vi "FG_registeredwindows.vi"(8 "error in (no error)":errorcluster, 10 "window":T2, 11 "action":T1) -> (0 "error out":errorcluster, 2 "windows":T2[](array[typedef]))   [LabVIEW 2009]
uses:
  child window props.ctl
  FG states.ctl
panel:
  in  "Error range offset":i32=5500
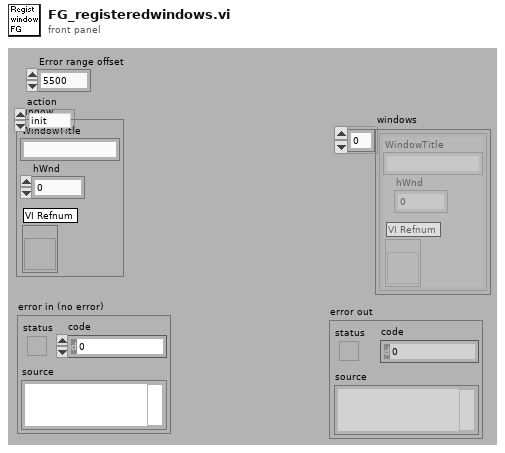
[diagram p1: front panel]
types:
  T1 = typedef "FG states.ctl" = enum16{"init", "add", "replace", "remove", "read"}
  T2 = typedef "child window props.ctl" = cluster{"WindowTitle":string, "hWnd":u32, "VI Refnum":refnum<vi>}
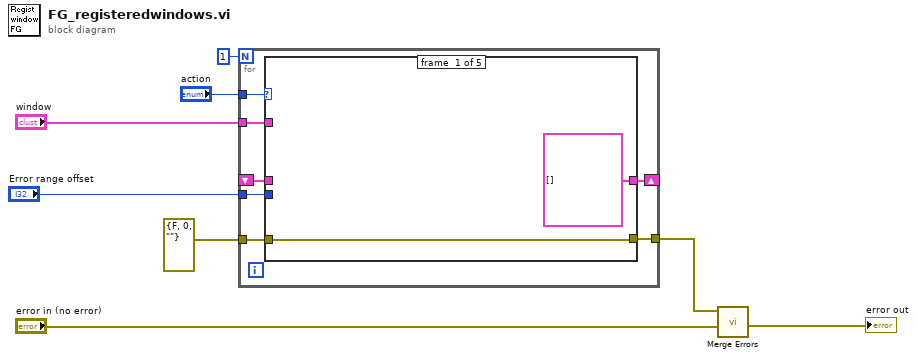
[diagram p0: block diagram]
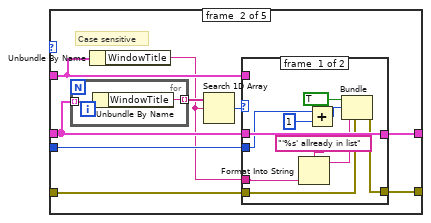
[diagram p2: hidden frame]
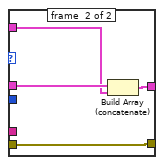
[diagram p3: hidden frame]
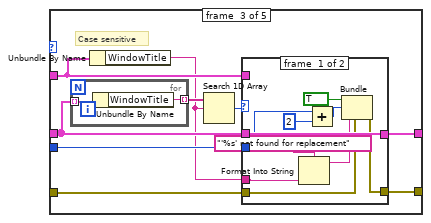
[diagram p4: hidden frame]
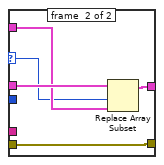
[diagram p5: hidden frame]
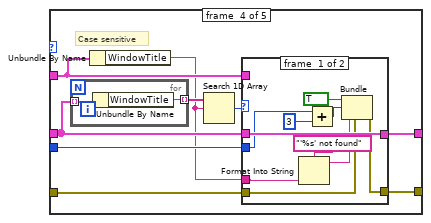
[diagram p6: hidden frame]
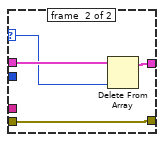
[diagram p7: hidden frame]
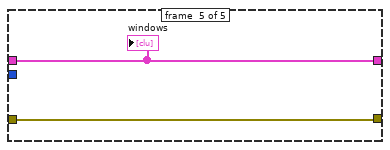
[diagram p8: hidden frame]
diagram:
  n1 = for {
    N: 1 -> [_]
    tunnel: "window" -> [w13]
    tunnel: "action" -> [w15]
    shift-right: [w12] -> _
    shift-left: _ -> [w14]
    tunnel: errorcluster {"status"=FALSE, "code"=0, "source"=""} ("error in (no error)") -> [w11]
    tunnel: [w10] -> w2
    tunnel: "Error range offset" -> [w9]
    n2 = case shown="\"init\", Default" w15 {
      tunnel: w14 -> [_ w25 w50 w76 w95]
      tunnel: w13 -> [_ w24 w49 w75 _]
      tunnel: [T2[] [] w26 w51 w77 w95] -> w12
      tunnel: w11 -> [w17 w21 w46 w72 w94]
      tunnel: [w17 w20 w45 w71 w94] -> w10
      tunnel: w9 -> [_ w19 w44 w70 _]
      frame #0 {
      }
      frame #1 {
        # "Case sensitive"
        n3 = for {
          tunnel: w25 -> [w42] mode=indexing
          tunnel: [w41] -> w23 mode=indexing
          n4 = Unbundle By Name(w42) -> ("WindowTitle"=w41:string)
        }
        n5 = Unbundle By Name(w24) -> ("WindowTitle"=w18:string)
        n6 = Search 1D Array(1D array=w23, element=w18) -> (index of element=w22:i32)  [unwired: 1 out]
        n7 = case shown="0, Default" w22 {
          tunnel: [w36 w40] -> w26
          tunnel: w25 -> [w36 w39]
          tunnel: w24 -> [_ w38]
          tunnel: w21 -> [w35 w37]
          tunnel: [w34 w37] -> w20
          tunnel: w19 -> [w32 _]
          tunnel: w18 -> [w29 _]
          frame #0 {
            n8 = Format Into String(format string="'%s' allready in list", w29) -> (resulting string=w28:string)  [unwired: 2 in, 1 out]
            n9 = Add(x=w32, y=1) -> (x+y=w31:i32)
            n10 = Bundle(cluster=w35, "status"=TRUE, "code"=w31, "source"=w28) -> (w34:errorcluster)
          }
          frame #1 {
            n11 = Build Array (concatenate)(w39, w38) -> (w40:T2[])
          }
        }
      }
      frame #2 {
        # "Case sensitive"
        n12 = for {
          tunnel: w50 -> [w68] mode=indexing
          tunnel: [w67] -> w48 mode=indexing
          n13 = Unbundle By Name(w68) -> ("WindowTitle"=w67:string)
        }
        n14 = Unbundle By Name(w49) -> ("WindowTitle"=w43:string)
        n15 = Search 1D Array(1D array=w48, element=w43) -> (index of element=w47:i32)  [unwired: 1 out]
        n16 = case shown="-1" w47 {
          selector: w47 -> [_ w62]
          tunnel: [w61 w66] -> w51
          tunnel: w50 -> [w61 w65]
          tunnel: w49 -> [_ w63]
          tunnel: w46 -> [w60 w64]
          tunnel: [w59 w64] -> w45
          tunnel: w44 -> [w57 _]
          tunnel: w43 -> [w54 _]
          frame #0 {
            n17 = Format Into String(format string="'%s' not found for replacement", w54) -> (resulting string=w53:string)  [unwired: 2 in, 1 out]
            n18 = Add(x=w57, y=2) -> (x+y=w56:i32)
            n19 = Bundle(cluster=w60, "status"=TRUE, "code"=w56, "source"=w53) -> (w59:errorcluster)
          }
          frame #1 {
            n20 = Replace Array Subset(array=w65, new element=w63, index=w62) -> (w66:T2[])
          }
        }
      }
      frame #3 {
        # "Case sensitive"
        n21 = for {
          tunnel: w76 -> [w93] mode=indexing
          tunnel: [w92] -> w74 mode=indexing
          n22 = Unbundle By Name(w93) -> ("WindowTitle"=w92:string)
        }
        n23 = Unbundle By Name(w75) -> ("WindowTitle"=w69:string)
        n24 = Search 1D Array(1D array=w74, element=w69) -> (index of element=w73:i32)  [unwired: 1 out]
        n25 = case shown="-1" w73 {
          selector: w73 -> [_ w88]
          tunnel: [w87 w91] -> w77
          tunnel: w76 -> [w87 w90]
          tunnel: w75 -> [_ _]
          tunnel: w72 -> [w86 w89]
          tunnel: [w85 w89] -> w71
          tunnel: w70 -> [w83 _]
          tunnel: w69 -> [w80 _]
          frame #0 {
            n26 = Format Into String(format string="'%s' not found", w80) -> (resulting string=w79:string)  [unwired: 2 in, 1 out]
            n27 = Add(x=w83, y=3) -> (x+y=w82:i32)
            n28 = Bundle(cluster=w86, "status"=TRUE, "code"=w82, "source"=w79) -> (w85:errorcluster)
          }
          frame #1 {
            n29 = Delete From Array(array=w90, index=w88) -> (array with subset deleted=w91:T2[])  [unwired: 1 in, 1 out]
          }
        }
      }
      frame #4 {
        "windows" <- w95
      }
    }
  }
  n30 = call <vilib>:"Merge Errors.vi"("error in 3 (no error)"="error in (no error)", "error in 1 (no error)"=w2) -> ("error out"=→"error out":errorcluster)  [unwired: 2 in, 3 out]
